vi "udp.vi"() -> ()   [LabVIEW 2019]
panel:
  out "结束时间":timestamp
  out "开始时间":timestamp
  in  "判断条件":string
  in  "监听超时时间，-1为一直监听":dbl
  in  "监听ip地址":string
  in  "监听端口":u16
  out "源地址":u32
  out "源端口":u16
  out "接收数据输出":string
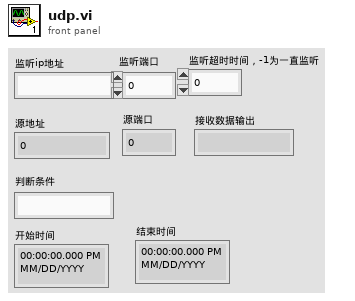
[diagram p1: front panel]
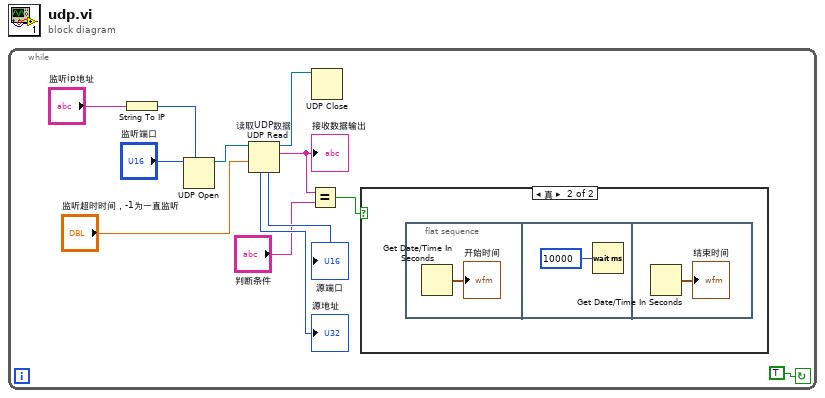
[diagram p0: block diagram]
diagram:
  n1 = while {
    stop <- TRUE continue-if-true
    n2 = String To IP(1:"监听ip地址") -> (0:w6:u32)
    n3 = UDP Open(7:w6, 11:"监听端口") -> (port=w10:refnum<k16>)  [unwired: 3 in, 2 out]
    n4 = UDP Read "读取UDP数据"(connection ID=w10, timeout ms (25000)="监听超时时间，-1为一直监听") -> (data out=w2:string, 3:w9:refnum<k16>, 4:→"源端口":u16, 6:→"源地址":u32)  [unwired: 2 in, 1 out]
    "接收数据输出" <- w2
    n5 = Equal?(x=w2, y="判断条件") -> (x = y?=w1:bool)
    n6 = UDP Close(connection ID=w9) -> ()  [unwired: 1 in, 2 out]
    n7 = case shown="真" w1 {
      frame False {
      }
      frame True {
        n8 = flat-sequence {
          frame #0 {
            n9 = Get Date/Time In Seconds() -> (seconds since 1Jan1904=→"开始时间":timestamp)
          }
          frame #1 {
            n10 = Wait (ms)(milliseconds to wait=u32 10000 ("毫秒计时值")) -> ()  [unwired: 1 out]
          }
          frame #2 {
            n11 = Get Date/Time In Seconds() -> (seconds since 1Jan1904=→"结束时间":timestamp)
          }
        }
      }
    }
  }
